vi "Get Output Values.vi"(0 "VISA resource name":refnum<visa-resource-name>, 11 "error in (no error)":errorcluster) -> (3 "Primary Value":dbl format="%^.3e", 4 "VISA resource name out":refnum<visa-resource-name>, 6 "Primary Value Units":i32, 8 "Secondary Value":dbl format="%^.3e", 10 "Secondary Value Units":i32, 14 "Fundamental Frequency":dbl format="%^.3e", 15 "error out":errorcluster)   [LabVIEW 2013, in "Fluke 5XXX Series Multicalibrators.lvlib"]
doc: "This VI returns the output amplitudes and frequency of the Calibrator.\n\nNote:\n\n(1) Instrument models 5700A, 5720A and 57LFC are not equipped with dual outpus. Only single output operations are available."
uses:
  Fluke 5XXX Series Multicalibrators.lvlib
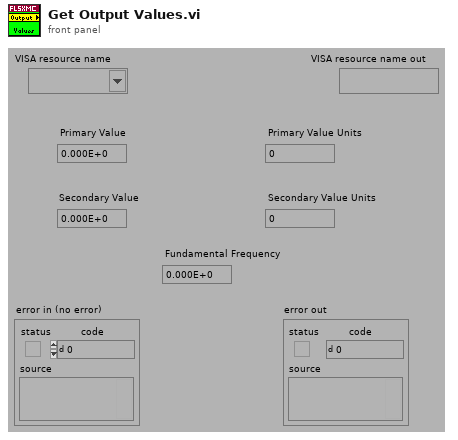
[diagram p1: front panel]
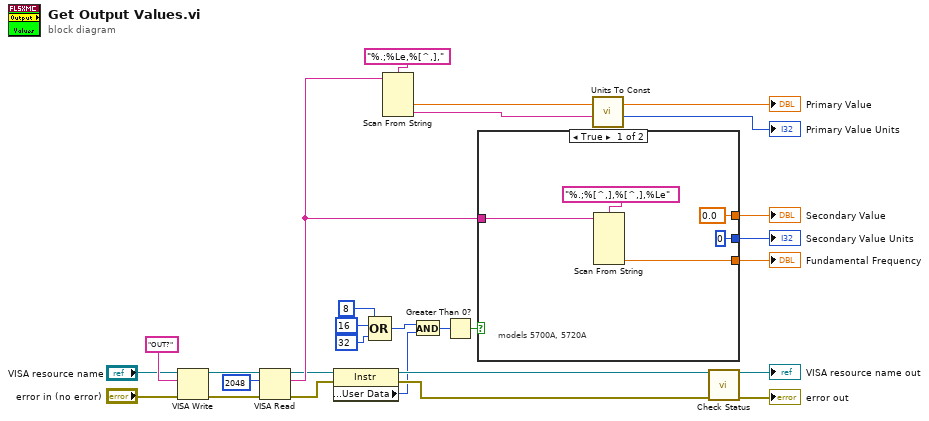
[diagram p0: block diagram]
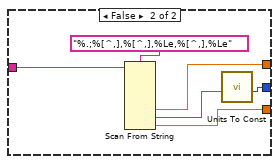
[diagram p2: hidden frame]
diagram:
  n1 = VISA Write(VISA resource name="VISA resource name", write buffer="OUT?", error in (no error)="error in (no error)") -> (VISA resource name out=w26:refnum<visa-resource-name>, error out=w25:errorcluster)  [unwired: 1 out]
  n2 = VISA Read(VISA resource name=w26, byte count=u32 2048 ("byte count (0)"), error in (no error)=w25) -> (VISA resource name out=w9:refnum<visa-resource-name>, read buffer=w13:string, error out=w7:errorcluster)  [unwired: 1 out]
  n3 = property class="Instr"(reference=w9, error in=w7) -> (reference out=w8:refnum<visa-resource-name>, error out=w6:errorcluster, "General Settings:User Data"=w5:u32)
  n4 = Compound Arithmetic op=OR(u32 8 ("Numeric"), u32 16 ("Numeric"), u32 32 ("Numeric")) -> (w4:u32)
  n5 = Scan From String(format string="%.;%Le,%[^,],", input string=w13) -> (output 1=→"Primary Value":dbl, output 2=w15:string)  [unwired: 4 in, 3 out]
  n6 = And(x=w4, y=w5) -> (x .and. y?=w3:u32)
  n7 = Greater Than 0?(x=w3) -> (x > 0?=w2:bool)
  n8 = case shown="True" w2 {
    tunnel: w13 -> [w31 w37]
    tunnel: [w30 w36] -> w12
    tunnel: [0 ("Const") w34] -> w11
    tunnel: [0.0 w33] -> w10
    frame True {
      # "models 5700A, 5720A"
      n9 = Scan From String(format string="%.;%[^,],%[^,],%Le" ("Format String"), input string=w31) -> (output 3=w30:dbl)  [unwired: 7 in, 3 out]
    }
    frame False {
      n10 = Scan From String(format string="%.;%[^,],%[^,],%Le,%[^,],%Le" ("Format String"), input string=w37) -> (output 3=w33:dbl, output 4=w35:string, output 5=w36:dbl)  [unwired: 9 in, 3 out]
      n11 = call "Units To Const.vi"("Units"=w35) -> ("Const"=w34:i32)  [unwired: 10 in]
    }
  }
  "Secondary Value" <- w10
  "Secondary Value Units" <- w11
  "Fundamental Frequency" <- w12
  n12 = call "Units To Const.vi"("Units"=w15) -> ("Const"=→"Primary Value Units":i32)  [unwired: 10 in]
  n13 = call "Check Status.vi"("VISA resource name"=w8, "error in (no error)"=w6) -> ("VISA resource name out"=→"VISA resource name out":refnum<visa-resource-name>, "error out"=→"error out":errorcluster)  [unwired: 12 in]
